vi "Arcade Drive.vi"(8 "Max Output":dbl, 10 "Y Axis":dbl, 11 "X Axis":dbl) -> (2 "Left Motor Value":dbl, 3 "Right Motor Value":dbl)   [LabVIEW 2012]
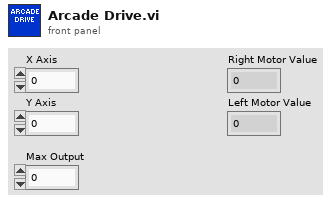
[diagram p1: front panel]
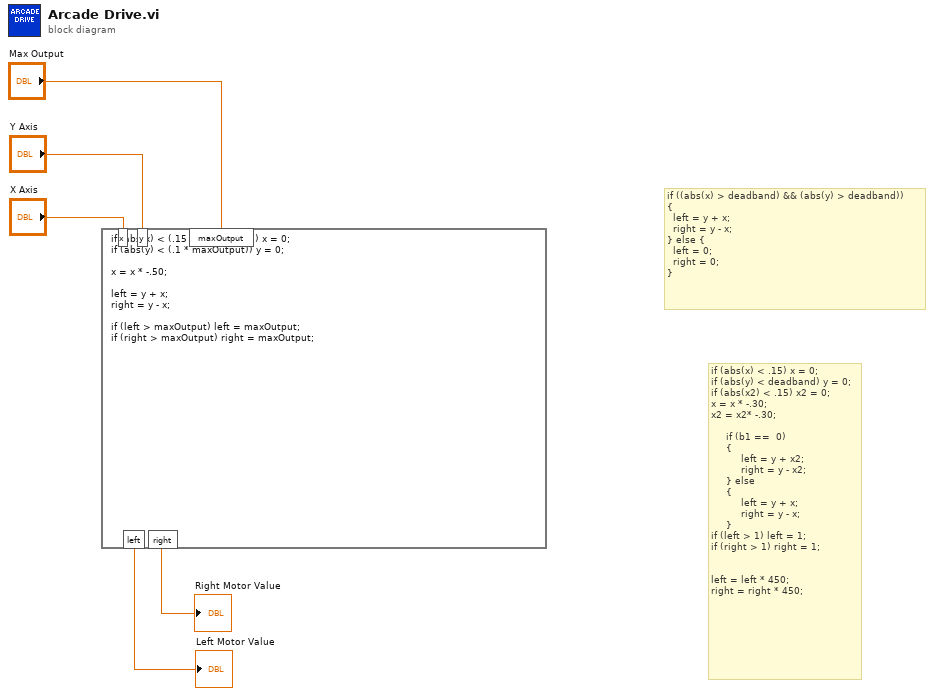
[diagram p0: block diagram]
diagram:
  # "if ((abs(x) > deadband) && (abs(y) > deadband))\n{\n  left = y + x;\n  right = y - x;\n} else {\n  left = 0;\n  right = 0;\n}"
  # "if (abs(x) < .15) x = 0;\nif (abs(y) < deadband) y = 0;\nif (abs(x2) < .15) x2 = 0;\nx = x * -.30;\nx2 = x2* -.30;\n\n     if (b1 ==  0)\n     {\n          left = y + x2;\n          right = y - x2;\n     } else\n     {\n          left = y + x;\n          right = y - x;\n     }\nif (left > 1) left = 1;\nif (right > 1) right = 1;\n\n\nleft = left * 450;\nright = right * 450;"
  n1 = formula code="if (abs(x) < (.15 * maxOutput)) x = 0;\nif (abs(y) < (.1 * maxOutput)) y = 0;\n\nx = x * -.50;\n\nleft = y + x;\nright = y - x;\n\nif (left > maxOutput) left = maxOutput;\nif (right > maxOutput) right = maxOutput;"("x"="X Axis", "y"="Y Axis", "maxOutput"="Max Output") -> ("left"=→"Left Motor Value":dbl, "right"=→"Right Motor Value":dbl)
